vi "Total Shift.vi"(11 "connection reference":T1) -> (0 "Total Shifts":i32, 2 "Shift Hrs":i32)   [LabVIEW 2017]
uses:
  <vilib>/addons/database/Connection.llb/Conn ObjectReference.ctl
  <vilib>/addons/database/Connection.llb/Conn Execute.vi
  <vilib>/addons/database/Recordset.llb/Rec Fetch Recordset Data (R).vi
  <vilib>/addons/database/Recordset.llb/Rec Destroy - Connection.vi
  <vilib>/addons/database/NI_Database_API.lvlib
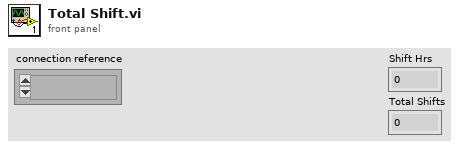
[diagram p1: front panel]
types:
  T1 = typedef "NI_Database_API.lvlib/Conn ObjectReference.ctl" = refnum<k1>
  T2 = typedef "NI_Database_API.lvlib/Rec ObjectReference.ctl" = refnum<k1>
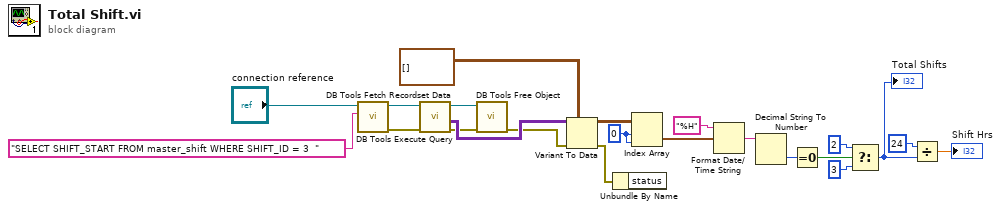
[diagram p0: block diagram]
diagram:
  w16 = 0 ("index (row)")
  n1 = call-poly <vilib>:"DB Tools Execute Query.vi"("SQL query"="SELECT SHIFT_START FROM master_shift WHERE SHIFT_ID = 3  ", "connection reference"="connection reference") -> ("error out"=w4:errorcluster, "recordset reference"=w21:T2)  [unwired: 6 in]
  n2 = call-poly <vilib>:"DB Tools Fetch Recordset Data.vi"("error in (no error)"=w4, "recordset reference"=w21) -> ("error out"=w2:errorcluster, "recordset data"=w20:variant[][], "recordset reference out"=w3:T2)  [unwired: 3 in]
  n3 = call-poly <vilib>:"DB Tools Free Object.vi"("error in (no error)"=w2, "recordset reference"=w3) -> ("error out"=w1:errorcluster)  [unwired: 8 in, 1 out]
  n4 = Variant To Data(error in=w1, type=timestamp[][] [] ("From Date 2"), Variant=w20) -> (data=w17:timestamp[][], error out=w5:errorcluster)
  n5 = Unbundle By Name(w5) -> ()  [unwired: 1 out]
  n6 = Index Array(array=w17, index (row)=w16, index (col)=w16) -> (element=w15:timestamp)
  n7 = Format Date/Time String(time format string (%c)="%H", seconds (now)=w15) -> (date/time string=w10:string)  [unwired: 1 in]
  n8 = Decimal String To Number(string=w10) -> (number=w9:i32)  [unwired: 2 in, 1 out]
  n9 = Equal To 0?(x=w9) -> (x = 0?=w11:bool)
  n10 = Select(t=2, s=w11, f=3) -> (s? t:f=w8:i32)
  "Total Shifts" <- w8
  n11 = Divide(x=24, y=w8) -> (x/y=→"Shift Hrs":dbl)
